vi "Filter.vi"(8 "X":dbl[](array[numeric]), 9 "N":dbl, 11 "tempdata in":dbl[][](array[numeric])) -> (0 "XFiltered":dbl[](array[numeric]), 3 "tempdata out":dbl[][](array[numeric]))   [LabVIEW 2011]
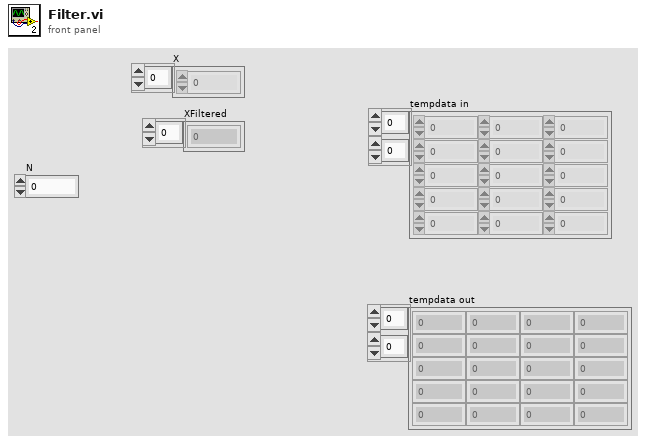
[diagram p1: front panel]
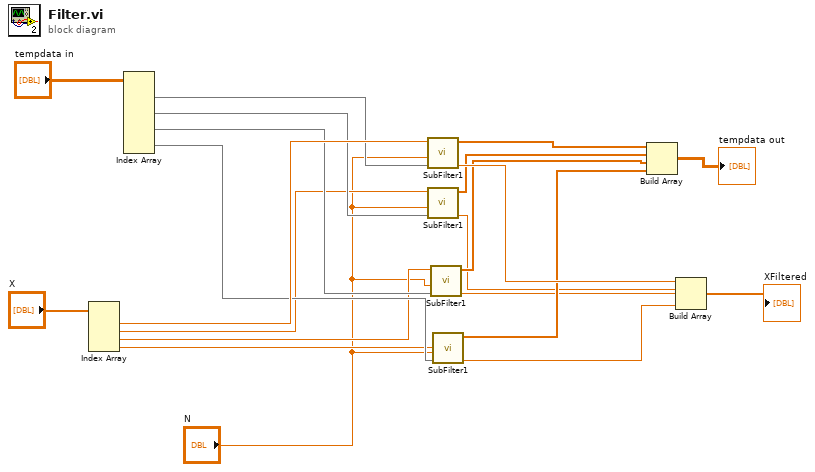
[diagram p0: block diagram]
diagram:
  n1 = Index Array(array="X") -> (element #1=w20:dbl, element #2=w10:dbl, element #3=w9:dbl, element #4=w8:dbl)  [unwired: 4 in]
  n2 = Index Array(array="tempdata in") -> (element #1=w15:dbl[], element #2=w13:dbl[], element #3=w12:dbl[], element #4=w11:dbl[])  [unwired: 8 in]
  n3 = call "SubFilter1.vi"("Array1"=w15, "N"="N", "X"=w20) -> ("XFiltered"=w19:dbl, "Array 2"=w17:dbl[])  [unwired: 7 in]
  n4 = call "SubFilter1.vi"("Array1"=w13, "N"="N", "X"=w10) -> ("XFiltered"=w4:dbl, "Array 2"=w7:dbl[])  [unwired: 7 in]
  n5 = call "SubFilter1.vi"("Array1"=w12, "N"="N", "X"=w9) -> ("XFiltered"=w3:dbl, "Array 2"=w6:dbl[])  [unwired: 7 in]
  n6 = call "SubFilter1.vi"("Array1"=w11, "N"="N", "X"=w8) -> ("XFiltered"=w2:dbl, "Array 2"=w5:dbl[])  [unwired: 7 in]
  n7 = Build Array(w17, w7, w6, w5) -> (→"tempdata out":dbl[][])
  n8 = Build Array(w19, w4, w3, w2) -> (→"XFiltered":dbl[])
